vi "Main.vi"(11 "Module Admin":refnum<class "Delacor_lib_QMH_Module Admin.lvclass">) -> ()   [LabVIEW 2020, in "Rename As Application UI.lvlib"]
doc: "This template is based off of the Queued Message Handler design pattern and the Queued Message Handler project template that ships with LabVIEW.\n\nThe main difference is that the queue is private to this module and communication between modules is performed via Broadcast and Request events.\n\nRequest events are wrapped in public API methods and are handled in the Event Handling Loop (EHL) of this VI. Any module can register for Broadcast events sent by this module. The EHL generates messages based on user interface actions.\n\nThe Message Handling Loop (MHL) processes messages generated by the EHL, or by other messages. The messages are string values, so new messages can be added easily to the Message Cases case structure in the MHL. Each message cluster can also provide an optional value for Message Data, which is a variant that can be converted to whatever message-specific data is required.\n_____\nBased on DQMH Project Template 6.1.0.94."
uses:
  Rename As Application UI.lvlib
  <vilib>/Delacor/Delacor QMH/Libraries/Module Admin_class/Delacor_lib_QMH_Module Admin.lvclass
  Module Data--cluster.ctl
  Configuration/Configuration--cluster.ctl
  <vilib>/Delacor/Delacor QMH/Libraries/Message Queue_class/Delacor_lib_QMH_Message Queue.lvclass/Delacor_lib_QMH_Message Queue.ctl
  Stop Argument--cluster.ctl
  <vilib>/Utility/miscctls.llb/LVPointTypeDef.ctl
  <vilib>/Delacor/Delacor QMH/Libraries/Module Admin_class/Delacor_lib_QMH_Module Admin.lvclass/Delacor_lib_QMH_Module Admin.ctl
  <vilib>/Delacor/Delacor QMH/Libraries/Message Queue_class/Delacor_lib_QMH_Enqueue Message (Single).vi
  <vilib>/Delacor/Delacor QMH/Libraries/Module Admin_class/Delacor_lib_QMH_Get External Launch.vi
  <vilib>/Utility/error.llb/Error Cluster From Error Code.vi
  <vilib>/ErrorRing/Error Ring.xnode
  <vilib>/Delacor/Delacor QMH/Libraries/Message Queue_class/Delacor_lib_QMH_Message Queue.lvclass
  <vilib>/Peloton/Pelobuttons/Pelobuttons_lib_Pelobuttons.lvlib
  Configuration/Configuration.lvlib
  <vilib>/Peloton/Peloton Config/Libraries/DCFG Framework/Peloton_DCFG Framework.lvlib
  Rename As Application Shared/Rename as Application Shared.lvlib
  Motherboard loading/Motherboard loading.lvlib
panel:
  in  "STOP":bool
  in  "Detecting speed":dbl caption="Detecting spedd" format="%#_6pms"
  in  "Start Acquisition":bool
  out "Waveform Chart":i32(graph)
  out "version":string
  in  "About":bool
  in  "Configuration":bool
  in  "Random Path":path
  out "error out":errorcluster
  in  "Simulate MHL Error":bool
  in  "Simulate EHL Error":bool
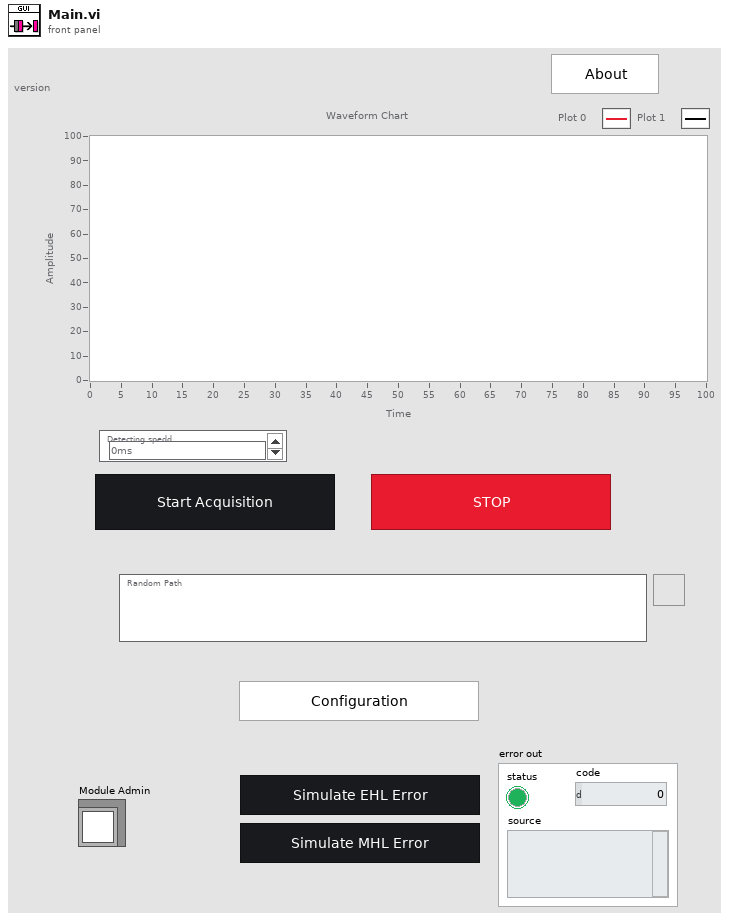
[diagram p1: front panel]
types:
  T1 = typedef "Rename As Application UI.lvlib/Request Events--cluster.ctl" = cluster{"Stop Module":refnum<user-event>, "Show Panel":refnum<user-event>, "Hide Panel":refnum<user-event>, "Get Module Execution Status":refnum<user-event>, "Show Diagram":refnum<user-event>}
  T2 = typedef "Peloton_DCFG Framework.lvlib/Broadcast Events--cluster.ctl" = cluster{"Module Did Init":refnum<user-event>, "Status Updated":refnum<user-event>, "Error Reported":refnum<user-event>, "Module Did Stop":refnum<user-event>, "Update Module Execution Status":refnum<user-event>, "View Changed":refnum<user-event>, "Configuration Updated":refnum<user-event>, "Page Error Received":refnum<user-event>, "Page List Updated":refnum<user-event>, "Defaults Applied":refnum<user-event>, "Main Window Closed":refnum<user-event>}
  T3 = typedef "Motherboard loading.lvlib/Broadcast Events--cluster.ctl" = cluster{"Module Did Init":refnum<user-event>, "Status Updated":refnum<user-event>, "Error Reported":refnum<user-event>, "Module Did Stop":refnum<user-event>, "Update Module Execution Status":refnum<user-event>, "CPU Loading updated":refnum<user-event>}
  T4 = typedef "Rename As Application UI.lvlib/Module Data--cluster.ctl" = cluster{"UI Configuration":T5}
  T5 = typedef "Rename As Application UI.lvlib/Configuration.lvlib/Configuration--cluster.ctl" = cluster{"Random Path":path}
  T6 = enum32{"invalid lock state", "Not Locked", "Locked (No Password)", "Password-protected"}
  T7 = typedef "Rename As Application UI.lvlib/Stop Argument--cluster.ctl" = cluster{"Origin":string, "Exit via Stop Module Req?":bool, "Wait for Module to stop?":bool}
  T8 = typedef "LVPointTypeDef.ctl" = cluster{"Horizontal":i16, "Vertical":i16}
  T9 = enum32{"Invalid", "Standard", "Closed", "Hidden", "Minimized", "Maximized"}
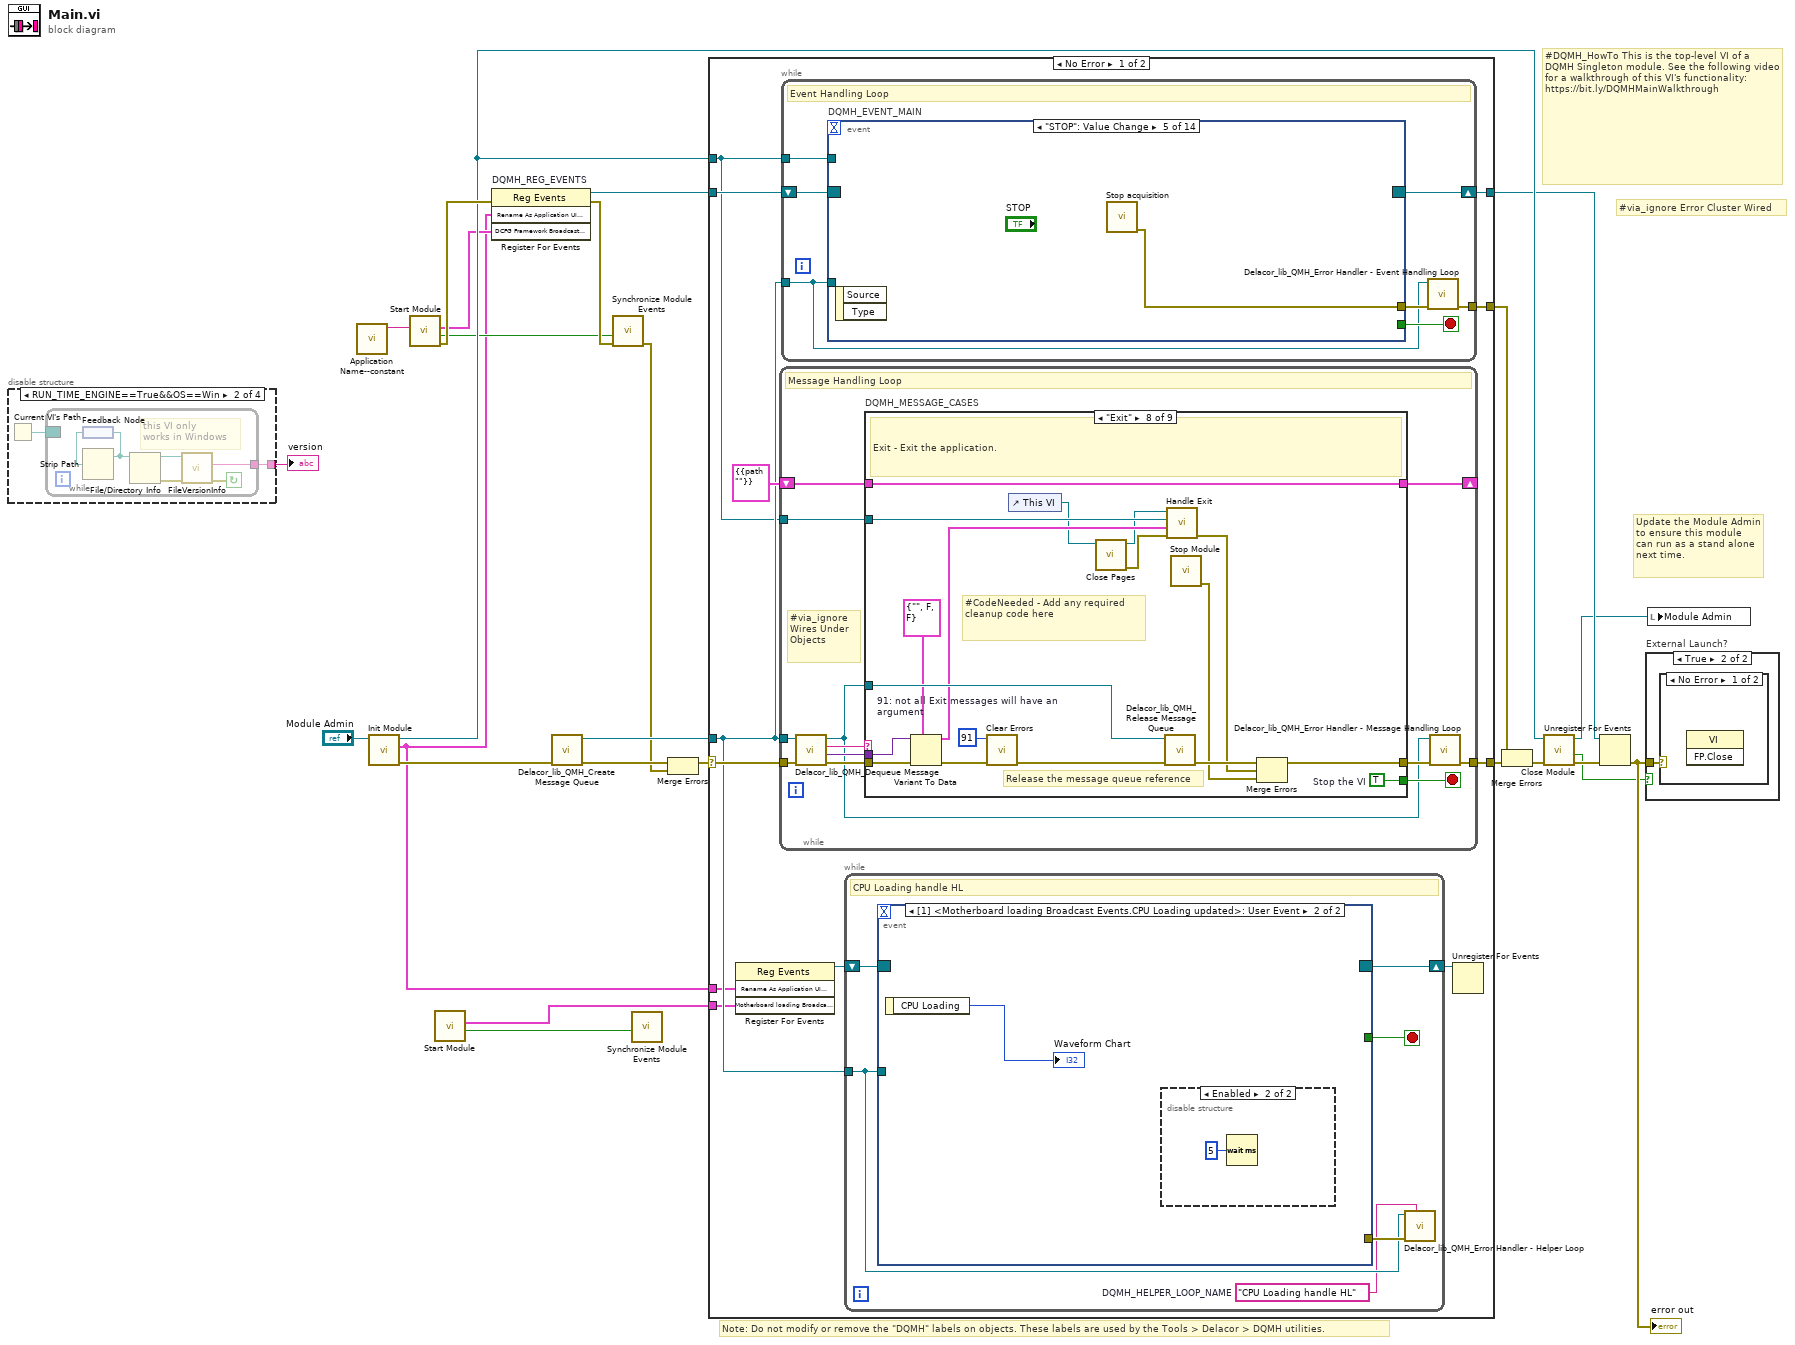
[diagram p0: block diagram]
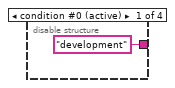
[diagram p2: hidden frame]
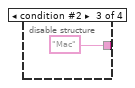
[diagram p3: hidden frame]
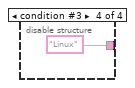
[diagram p4: hidden frame]
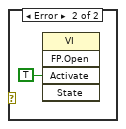
[diagram p6: hidden frame]
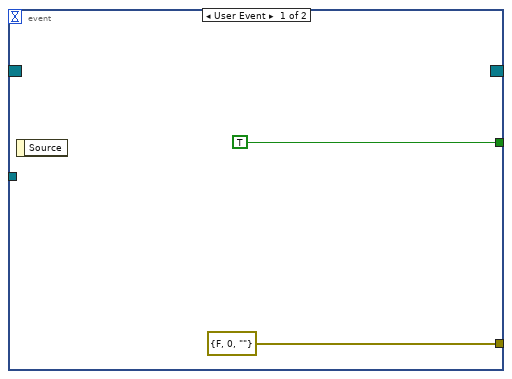
[diagram p7: hidden frame]
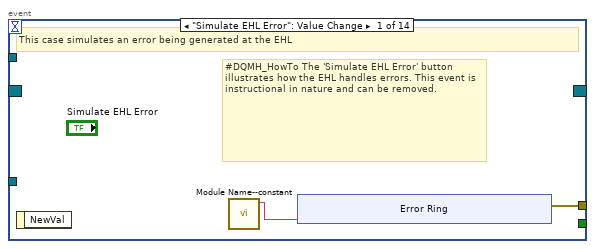
[diagram p9: hidden frame]
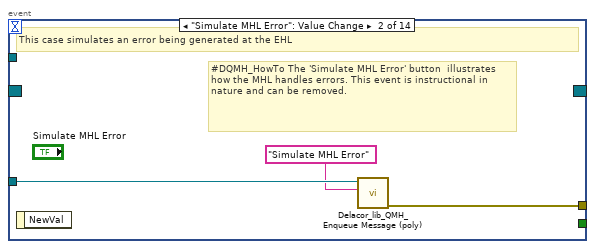
[diagram p10: hidden frame]
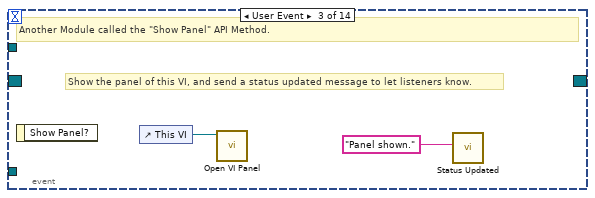
[diagram p11: hidden frame]
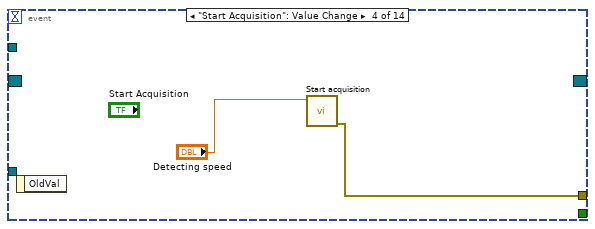
[diagram p12: hidden frame]
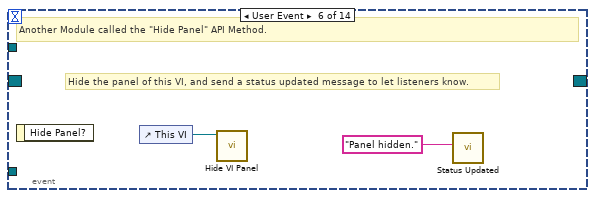
[diagram p13: hidden frame]
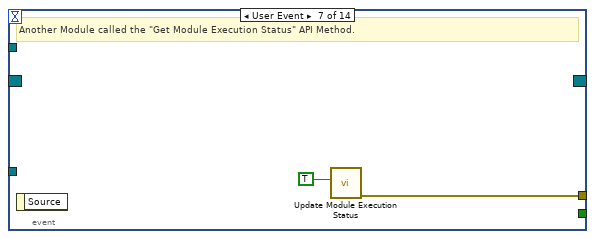
[diagram p14: hidden frame]
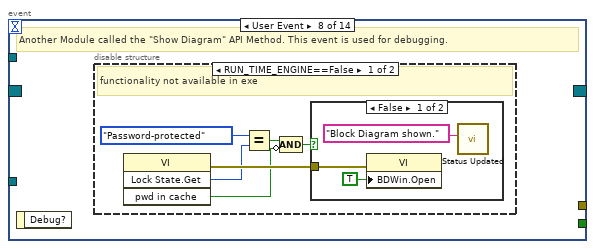
[diagram p15: hidden frame]
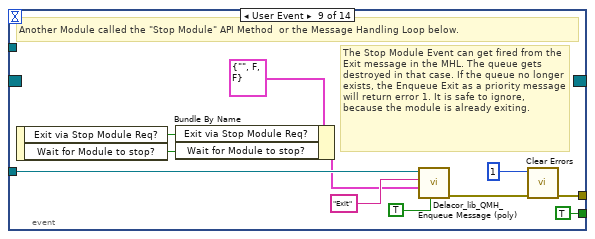
[diagram p18: hidden frame]
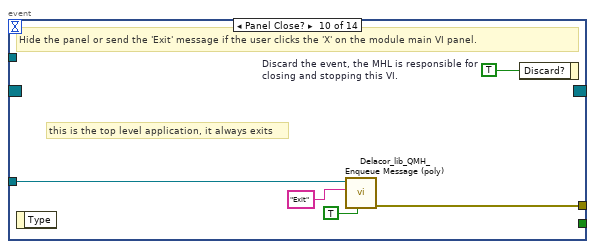
[diagram p19: hidden frame]
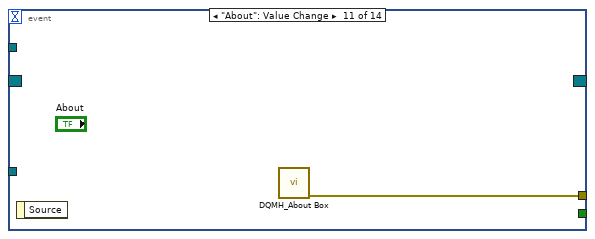
[diagram p20: hidden frame]
diagram:
  # "#via_ignore Error Cluster Wired"
  # "#DQMH_HowTo This is the top-level VI of a DQMH Singleton module. See the following video for a walkthrough of this VI's functionality: https://bit.ly/DQMHMainWalkthrough"
  # "Note: Do not modify or remove the \"DQMH\" labels on objects. These labels are used by the Tools > Delacor > DQMH utilities."
  # "Update the Module Admin to ensure this module can run as a stand alone next time."
  n1 = disable-structure "Conditional Disable Structure" shown="RUN_TIME_ENGINE==True&&OS==Win" {
    disable-tunnel: ["development" w27 "Mac" "Linux"] -> w4
    frame condition #0 (active) {
    }
    frame condition #1 {
      n2 = Current VI's Path() -> (path=w28:path)
      n3 = while {
        border: w28 -> [_]
        tunnel: [w29] -> w27
        stop <- w33 continue-if-true
        # "this VI only \nworks in Windows"
        n4 = feedback #1() -> (w32:path)
        n5 = Strip Path(path=w32) -> (stripped path=w31:path)  [unwired: 1 out]
        n6 = feedback-in #1(w31) -> ()
        n7 = File/Directory Info(path=w31) -> (path out=w30:path, error out=w34:errorcluster)  [unwired: 1 in, 5 out]
        n8 = call <vilib>:"FileVersionInfo.vi"("error in (no error)"=w34, "Application Path in"=w30) -> ("error out"=w33:errorcluster, "File Version Info"=w29:string)  [unwired: 6 in, 2 out]
      }
    }
    frame condition #2 {
    }
    frame condition #3 {
    }
  }
  "version" <- w4
  n9 = call "Application Name--constant.vi"() -> ("Application Name"=w9:string)  [unwired: 11 in]
  n10 = call "Init Module.vi"("Singleton Module Admin in"="Module Admin") -> ("error out"=w23:errorcluster, "Rename As Application UI Request Events"=w2:T1, "Singleton Module Admin out"=w16:refnum<class "Delacor_lib_QMH_Module Admin.lvclass">)  [unwired: 8 in]
  n11 = call <vilib>:"Start Module.vi"("Application Name"=w9) -> ("error out"=w25:errorcluster, "Wait for Event Sync?"=w6:bool, "DCFG Framework Broadcast Events"=w5:T2)  [unwired: 7 in, 1 out]
  n12 = call <vilib>:"Start Module.vi"() -> ("Wait for Event Sync?"=w3:bool, "Motherboard loading Broadcast Events"=w1:T3)  [unwired: 8 in, 2 out]
  n13 = register-events "DQMH_REG_EVENTS"(error in=w25, w2, w5) -> (reference out=w14:refnum<event-registration>, error out=w8:errorcluster)  [unwired: 1 in]
  n14 = call <vilib>:"Delacor_lib_QMH_Create Message Queue.vi"("error in"=w23) -> ("error out"=w18:errorcluster, "Message Queue"=w13:refnum<class "Delacor_lib_QMH_Message Queue.lvclass">)  [unwired: 9 in]
  n15 = call <vilib>:"Synchronize Module Events.vi"("error in (no error)"=w8, "Wait for Event Sync?"=w6) -> ("error out"=w7:errorcluster)  [unwired: 9 in]
  n16 = call <vilib>:"Synchronize Module Events.vi"("Wait for Event Sync?"=w3) -> ()  [unwired: 10 in, 1 out]
  n17 = Merge Errors(w18, w7) -> (w17:errorcluster)
  n18 = case shown="No Error" w17 {
    selector: w17 -> [w46 w235]
    tunnel: [w48 w234] -> w24
    tunnel: [w45 w240] -> w15
    tunnel: w14 -> [w43 w240]
    tunnel: w13 -> [w42 w233]
    tunnel: [w47 _] -> w21
    tunnel: w16 -> [w41 w236]
    tunnel: w2 -> [w40 _]
    tunnel: w1 -> [w37 _]
    frame No Error {
      n19 = register-events ("DQMH_HELPER_REGFOREVENTS")(w40, w37) -> (reference out=w38:refnum<event-registration>)  [unwired: 2 in, 1 out]
      n20 = while {
        tunnel: w42 -> [w127]
        shift-right: [w131] -> _
        shift-left: T4 {"UI Configuration"={"Random Path"=path ""}} ("Data Cluster") -> [w132]
        tunnel: w46 -> [w135]
        tunnel: [w133] -> w48
        tunnel: w41 -> [w125]
        stop <- w130 stop-if-true
        # "#via_ignore Wires Under Objects"
        # "Message Handling Loop"
        n21 = call-dynamic "Delacor_lib_QMH_Dequeue Message.vi"("error in"=w135, "Message Queue in"=w127) -> ("error out"=w134:errorcluster, "Message Data"=w128:variant, "Message"=w129:string, "Message Queue out"=w126:refnum<class "Delacor_lib_QMH_Message Queue.lvclass">)  [unwired: 6 in]
        n22 = case "DQMH_MESSAGE_CASES" shown="\"Exit\"" w129 {
          selector: w129 -> [_ _ _ _ _ _ _ _ w220]
          tunnel: w126 -> [_ _ _ _ _ _ w187 w211 _]
          tunnel: w134 -> [w155 w159 w167 w170 w172 w177 w194 w217 w222]
          tunnel: [w154 w159 w164 w169 w172 w176 w190 w214 w223] -> w136
          tunnel: w132 -> [w145 w158 w166 w168 w171 w174 w189 w210 w221]
          tunnel: [w144 w158 w165 w168 w171 w174 w189 w210 w221] -> w131
          tunnel: [_ _ _ _ _ _ _ w209 _] -> w130
          tunnel: w128 -> [_ _ w163 _ _ _ w188 w218 _]
          tunnel: w125 -> [w146 _ _ _ _ _ w186 w205 _]
          frame "Initialize" {
            # "#CodeNeeded - Initialize the appearance of the front panel."
            # "Initialize - Any operation that needs to be done before the module can receive messages. Synchronize Caller Events.vi will inform Start Module.vi that the module has launched and is ready to receive messages. Module Did Init.vi will broadcast that the module initialized."
            n23 = call "Synchronize Caller Events.vi"("error in (no error)"=w155, "Singleton Module Admin in"=w146) -> ("error out"=w139:errorcluster, "Singleton Module Admin out"=w141:refnum<class "Delacor_lib_QMH_Module Admin.lvclass">)  [unwired: 8 in]
            n24 = property on="Property Node" class="Module Admin"(reference=w141) -> ("Accessors:External Launch"=w150:bool)  [unwired: 1 in, 2 out]
            n25 = flat-sequence {
              tunnel: w139 -> [_]
              frame #0 {
                n26 = call <vilib>:"Brand UI - FP.vi"() -> ()  [unwired: 12 in]
              }
            }
            n27 = call "Add Pages.vi"("error in (no error)"=w139) -> ("latest data"=w138:T5)  [unwired: 9 in, 1 out]
            n28 = Select(t=T9."Hidden" ("State"), s=w150, f=T9."Standard" ("State")) -> (s? t:f=w147:T9)
            n29 = Unbundle By Name(w138) -> ("Random Path"=w137:path)
            n30 = call "Module Name--constant.vi"() -> ("Module Name"=w153:string)  [unwired: 11 in]
            n31 = property on="Property Node" class="VI"("Front Panel.Title"=w153) -> (reference out=w152:refnum<vi>, error out=w157:errorcluster)  [unwired: 2 in]
            n32 = call "Module Name--constant.vi"() -> ("Module Name"=w142:string)  [unwired: 11 in]
            n33 = local write "Random Path"(w137) -> ()
            n34 = Bundle By Name(cluster=w145, "UI Configuration"=w138) -> (w144:T4)
            n35 = invoke on="Invoke Node" class="VI" method="FP.Open"(reference=w152, error in=w157, "State"=w147) -> (reference out=w151:refnum<vi>, error out=w156:errorcluster)  [unwired: 2 in, 3 out]
            n36 = call "Module Did Init.vi"("error in (no error)"=w139, "Initialized?"=TRUE, "Origin"=w142) -> ("error out"=w154:errorcluster)  [unwired: 8 in]
            n37 = invoke on="Invoke Node" class="VI" method="FP.Center"(reference=w151, error in=w156) -> ()  [unwired: 1 in, 3 out]
            n38 = property on="Pane" class="Pane"("Origin"=T8 {"Horizontal"=0, "Vertical"=0}) -> ()  [unwired: 2 in, 2 out]
          }
          frame "---Module Specific---" {
            # "Separator -- The following cases handle messages specific to this Module."
          }
          frame "Configuration Updated" {
            # "The Configuration Editor has broadcasted that the Configuration has been updated"
            n39 = Variant To Data(error in=w167, type=T5 {"Random Path"=path ""} ("UI Configuration"), Variant=w163) -> (data=w161:T5, error out=w164:errorcluster)
            n40 = Unbundle By Name(w161) -> ("Random Path"=w160:path)
            n41 = Bundle By Name(cluster=w166, "UI Configuration"=w161) -> (w165:T4)
            n42 = local write "Random Path"(w160) -> ()
          }
          frame "---Copy This Frame---" {
            # "Duplicate this frame when creating new messages.  Change this comment in the duplicated frame to describe this message."
            n43 = Merge Errors(w170) -> (w169:errorcluster)
          }
          frame "---Exit and Error Handling---" {
            # "Separator - The following cases handle errors and exit messages."
          }
          frame "Simulate MHL Error" {
            # "#DQMH_HowTo The 'Simulate MHL Error' button  illustrates how the MHL handles errors. This event is instructional in nature and can be removed."
            # "Simulate an error occurring at the MHL"
            n44 = call "Module Name--constant.vi"() -> ("Module Name"=w173:string)  [unwired: 11 in]
            n45 = xnode ("Error Ring")("parameter 0"=w173) -> ("error out"=w175:errorcluster)
            n46 = Merge Errors(w177, w175) -> (w176:errorcluster)
          }
          frame "Error" {
            # "#CodeRecommended - If you ever change the name of this \"Error\" message, you'll need to update the name in the Check Loop Error.vi as well."
            # "#CodeRecommended - If the module is running in standalone mode (External Launch = FALSE), this code will pop up an error dialog and call the 'Exit' message if an error occurs. Add more fine-grained error handling here."
            # "Error - Check the error message data and respond accordingly. This message is sent by the \"Error Handler\" VIs at the end of each loop in this application."
            n47 = property on="Property Node" class="Module Admin"(reference=w186) -> ("Accessors:External Launch"=w185:bool)  [unwired: 1 in, 2 out]
            n48 = Variant To Data(error in=w194, type=errorcluster {"status"=FALSE, "code"=0, "source"=""} ("error constant"), Variant=w188) -> (data=w195:errorcluster, error out=w192:errorcluster)
            n49 = call "Error Reported.vi"("Error"=w195) -> ()  [unwired: 10 in, 1 out]
            n50 = case shown="False" w185 {
              tunnel: [w200 _] -> w191
              tunnel: w187 -> [w198 _]
              tunnel: w195 -> [w199 _]
              frame False {
                # "If the module is running standalone, then pop up an error dialog and call the \"Exit\" message."
                n51 = call <vilib>:"Simple Error Handler.vi"("error in (no error)"=w199) -> ()  [unwired: 4 in, 5 out]
                n52 = call-poly <vilib>:"Delacor_lib_QMH_Enqueue Message (poly).vi"("Priority Message? (F)"=TRUE, "Message"="Exit", "Message Queue in"=w198) -> ("error out"=w200:errorcluster)  [unwired: 7 in, 1 out]
              }
              frame True {
                # "If the module was launched externally, calling the Error Reported broadcast VI is the only action performed by the \"Error\" message. The module's caller can then process the error appropriately."
              }
            }
            n53 = Merge Errors(w192, w191) -> (w190:errorcluster)
            n54 = local write "error out"(w190) -> ()
          }
          frame "Exit" {
            w208 = 91  # 91: not all Exit messages will have an argument
            w209 = TRUE  # Stop the VI
            # "Release the message queue reference"
            # "#CodeNeeded - Add any required cleanup code here"
            # "Exit - Exit the application."
            n55 = Variant To Data(error in=w217, type=T7 {"Origin"="", "Exit via Stop Module Req?"=FALSE, "Wait for Module to stop?"=FALSE} ("Stop Argument"), Variant=w218) -> (data=w206:T7, error out=w213:errorcluster)
            n56 = call <vilib>:"Clear Errors.vi"("error in (no error)"=w213, "specific error code to clear (0: all)"=w208) -> ("error out"=w216:errorcluster)  [unwired: 4 in, 1 out]
            n57 = control-ref of="This VI"() -> (w203:refnum<vi>)
            n58 = call "Close Pages.vi"("Calling VI in"=w203) -> ("error out"=w204:errorcluster, "Calling VI out"=w202:refnum<vi>)  [unwired: 9 in]
            n59 = call-dynamic "Delacor_lib_QMH_Release Message Queue.vi"("error in"=w216, "Message Queue"=w211) -> ("error out"=w215:errorcluster)  [unwired: 9 in]
            n60 = call "Handle Exit.vi"("error in (no error)"=w204, "Stop Argument"=w206, "Admin in"=w205, "VI reference"=w202) -> ("error out"=w212:errorcluster)  [unwired: 6 in, 1 out]
            n61 = call "Stop Module.vi"() -> ("error out"=w201:errorcluster)  [unwired: 11 in]
            n62 = Merge Errors(w215, w212, w201) -> (w214:errorcluster)
          }
          frame Default {
            # "'Default' case only runs if there is a message that isn't defined in any of the other cases.  Output a programming error."
            n63 = call "Module Name--constant.vi"() -> ("Module Name"=w219:string)  [unwired: 11 in]
            n64 = xnode ("Error Ring")("parameter 0"=w220, "parameter 1"=w219) -> ("error out"=w224:errorcluster)
            n65 = Merge Errors(w222, w224) -> (w223:errorcluster)
          }
        }
        n66 = call-dynamic "Delacor_lib_QMH_Error Handler - Message Handling Loop.vi"("error in"=w136, "Message Queue in"=w126) -> ("dup error in"=w133:errorcluster)  [unwired: 8 in, 1 out]
      }
      n67 = while {
        tunnel: w42 -> [w59]
        shift-right: [w62] -> w45
        shift-left: w43 -> [w63]
        tunnel: [w64] -> w47
        tunnel: w41 -> [w60]
        stop <- w61 stop-if-true
        # "Event Handling Loop"
        n68 = event "DQMH_EVENT_MAIN" shown="[4] \"STOP\": Value Change" {
          selector: w63 -> [_ _ _ _ _ _ _ _ _ _ _ _ _ _]
          dyn-events: [_ _ _ _ _ _ _ _ _ _ _ _ _ _] -> w62
          timeout: _ -> [_ _ _ _ _ _ _ _ _ _ _ _ _ _]
          tunnel: [_ _ _ _ _ _ _ _ TRUE ("Discard?") _ _ _ _ _] -> w61
          tunnel: w59 -> [_ w76 _ _ _ _ _ _ w102 w109 _ _ w115 _]
          tunnel: [w67 w77 _ w81 w82 _ w86 _ w105 w111 w112 _ w114 w123] -> w65
          tunnel: w60 -> [_ _ _ _ _ _ _ _ _ _ _ _ _ _]
          event "Simulate EHL Error": Value Change {
            # "#DQMH_HowTo The 'Simulate EHL Error' button  illustrates how the EHL handles errors. This event is instructional in nature and can be removed."
            # "This case simulates an error being generated at the EHL"
            n69 = event-data() -> ()  [unwired: 1 in, 1 out]
            n70 = call "Module Name--constant.vi"() -> ("Module Name"=w66:string)  [unwired: 11 in]
            n71 = xnode ("Error Ring")("parameter 0"=w66) -> ("error out"=w67:errorcluster)
          }
          event "Simulate MHL Error": Value Change {
            # "#DQMH_HowTo The 'Simulate MHL Error' button  illustrates how the MHL handles errors. This event is instructional in nature and can be removed."
            # "This case simulates an error being generated at the EHL"
            n72 = event-data() -> ()  [unwired: 1 in, 1 out]
            n73 = call-poly <vilib>:"Delacor_lib_QMH_Enqueue Message (poly).vi"("Message"="Simulate MHL Error", "Message Queue in"=w76) -> ("error out"=w77:errorcluster)  [unwired: 8 in, 1 out]
          }
          event User Event {
            # "Show the panel of this VI, and send a status updated message to let listeners know."
            # "Another Module called the \"Show Panel\" API Method."
            n74 = event-data() -> ()  [unwired: 1 in, 1 out]
            n75 = control-ref of="This VI"() -> (w79:refnum<vi>)
            n76 = call "Open VI Panel.vi"("VI"=w79) -> ()  [unwired: 10 in, 1 out]
            n77 = call "Status Updated.vi"("Status"="Panel shown." ("format string")) -> ()  [unwired: 10 in, 1 out]
          }
          event "Start Acquisition": Value Change {
            n78 = event-data() -> ()  [unwired: 1 in, 1 out]
            n79 = call "Start acquisition.vi"("Detecting speed"="Detecting speed") -> ("error out"=w81:errorcluster)  [unwired: 9 in, 1 out]
          }
          event "STOP": Value Change {
            n80 = event-data() -> ()  [unwired: 1 in, 2 out]
            n81 = call "Stop acquisition.vi"() -> ("error out"=w82:errorcluster)  [unwired: 11 in]
          }
          event User Event {
            # "Hide the panel of this VI, and send a status updated message to let listeners know."
            # "Another Module called the \"Hide Panel\" API Method."
            n82 = event-data() -> ()  [unwired: 1 in, 1 out]
            n83 = control-ref of="This VI"() -> (w84:refnum<vi>)
            n84 = call "Hide VI Panel.vi"("VI"=w84) -> ()  [unwired: 10 in, 1 out]
            n85 = call "Status Updated.vi"("Status"="Panel hidden." ("format string")) -> ()  [unwired: 10 in, 1 out]
          }
          event User Event {
            # "Another Module called the \"Get Module Execution Status\" API Method."
            n86 = event-data() -> ()  [unwired: 1 in, 1 out]
            n87 = call "Update Module Execution Status.vi"("Running?"=TRUE) -> ("error out"=w86:errorcluster)  [unwired: 10 in]
          }
          event User Event {
            # "Another Module called the \"Show Diagram\" API Method. This event is used for debugging."
            n88 = event-data() -> ()  [unwired: 1 in, 1 out]
            n89 = disable-structure shown="RUN_TIME_ENGINE==False" {
              frame condition #0 (active) {
                # "functionality not available in exe"
                n90 = invoke on="Invoke Node" class="VI" method="Lock State.Get"() -> (error out=w92:errorcluster, "Get Lock State"=w91:T6, "pwd in cache"=w88:bool)  [unwired: 4 in, 1 out]
                n91 = Equal?(x=T6."Password-protected", y=w91) -> (x = y?=w89:bool)
                n92 = Compound Arithmetic op=AND(w89, invert w88) -> (w87:bool)
                n93 = case shown="False" w87 {
                  tunnel: w92 -> [w95 _]
                  frame False {
                    n94 = property on="Property Node" class="VI"(error in=w95, "BDWin.Open"=TRUE ("Block Diagram Window:Open")) -> ()  [unwired: 1 in, 2 out]
                    n95 = call "Status Updated.vi"("Status"="Block Diagram shown." ("format string")) -> ()  [unwired: 10 in, 1 out]
                  }
                  frame True {
                    # "Password-protected VI, and the password is not in the cache. Do not show the diagram."
                  }
                }
              }
              frame condition #1 {
              }
            }
          }
          event User Event {
            # "The Stop Module Event can get fired from the Exit message in the MHL. The queue gets destroyed in that case. If the queue no longer exists, the Enqueue Exit as a priority message will return error 1. It is safe to ignore, because the module is already exiting."
            # "Another Module called the \"Stop Module\" API Method  or the Message Handling Loop below."
            n96 = event-data() -> ("Exit via Stop Module Req?"=w98:bool, "Wait for Module to stop?"=w97:bool)  [unwired: 1 in]
            n97 = Bundle By Name(cluster=T7 {"Origin"="", "Exit via Stop Module Req?"=FALSE, "Wait for Module to stop?"=FALSE} ("Stop Argument"), "Exit via Stop Module Req?"=w98, "Wait for Module to stop?"=w97) -> (w96:T7)
            n98 = call-poly <vilib>:"Delacor_lib_QMH_Enqueue Message (poly).vi"("Priority Message? (F)"=TRUE, "Message Data"=w96, "Message"="Exit", "Message Queue in"=w102) -> ("error out"=w106:errorcluster)  [unwired: 6 in, 1 out]
            n99 = call <vilib>:"Clear Errors.vi"("error in (no error)"=w106, "specific error code to clear (0: all)"=1) -> ("error out"=w105:errorcluster)  [unwired: 4 in, 1 out]
          }
          event Panel Close? {
            w110 = TRUE  # Discard the event, the MHL is responsible for closing and stopping this VI.
            # "this is the top level application, it always exits"
            # "Hide the panel or send the 'Exit' message if the user clicks the 'X' on the module main VI panel."
            n100 = event-data() -> ()  [unwired: 1 in, 1 out]
            n101 = call-poly <vilib>:"Delacor_lib_QMH_Enqueue Message (poly).vi"("Priority Message? (F)"=TRUE, "Message"="Exit", "Message Queue in"=w109) -> ("error out"=w111:errorcluster)  [unwired: 7 in, 1 out]
            n102 = event-data ("Event Filter Node")("Discard?"=w110) -> ()  [unwired: 1 in, 1 out]
          }
          event "About": Value Change {
            n103 = event-data() -> ()  [unwired: 1 in, 1 out]
            n104 = call <vilib>:"DQMH_About Box.vi"() -> ("error out"=w112:errorcluster)  [unwired: 11 in]
          }
          event "Configuration": Value Change {
            n105 = event-data() -> ()  [unwired: 1 in, 1 out]
            n106 = call <vilib>:"Show Panel.vi"() -> ()  [unwired: 11 in, 1 out]
          }
          event User Event {
            # "The Configuration Editor has broadcasted that the Configuration has been updated"
            n107 = event-data() -> ("New Data"=w118:variant, "Name"=w117:string)  [unwired: 1 in]
            n108 = call "Handle Configuration Updated.vi"("Name"=w117, "New Data"=w118) -> ("Addressed to this Module"=w116:bool, "Latest Data"=w113:T5)  [unwired: 7 in, 1 out]
            n109 = case shown="True" w116 {
              tunnel: w115 -> [_ w122]
              tunnel: [_ w121] -> w114
              tunnel: w113 -> [_ w120]
              frame False {
              }
              frame True {
                n110 = call-poly <vilib>:"Delacor_lib_QMH_Enqueue Message (poly).vi"("Message Data"=w120, "Message"="Configuration Updated", "Message Queue in"=w122) -> ("error out"=w121:errorcluster)  [unwired: 7 in, 1 out]
              }
            }
          }
          event "Random Path": Value Change {
            n111 = event-data() -> ("NewVal"=w124:path)  [unwired: 1 in]
            n112 = call "Update Configuration.vi"("Random Path"=w124) -> ("error out"=w123:errorcluster)  [unwired: 10 in]
          }
        }
        n113 = call-dynamic "Delacor_lib_QMH_Error Handler - Event Handling Loop.vi"("error in"=w65, "Message Queue in"=w59) -> ("dup error in"=w64:errorcluster)  [unwired: 8 in, 1 out]
      }
      n114 = while "DQMH_HELPER_LOOP" {
        shift-right: [w53] -> w39
        shift-left: w38 -> [w54]
        tunnel: w42 -> [w50]
        stop <- w52 stop-if-true
        w49 = "CPU Loading handle HL"  # DQMH_HELPER_LOOP_NAME
        # "CPU Loading handle HL"
        n115 = event "DQMH_HELPER_EVENT_STRUCTURE" shown="[1] <Motherboard loading Broadcast Events.CPU Loading updated>: User Event" {
          selector: w54 -> [_ _]
          dyn-events: [_ _] -> w53
          timeout: _ -> [_ _]
          tunnel: [TRUE _] -> w52
          tunnel: [errorcluster {"status"=FALSE, "code"=0, "source"=""} ("error constant") _] -> w51
          tunnel: w50 -> [_ _]
          event User Event {
            n116 = event-data() -> ()  [unwired: 1 in, 1 out]
          }
          event User Event {
            n117 = event-data() -> ("CPU Loading"=→"Waveform Chart":i32)  [unwired: 1 in]
            n118 = disable-structure shown="Enabled" {
              frame Disabled {
              }
              frame Enabled {
                n119 = Wait (ms)(milliseconds to wait=u32 5) -> ()  [unwired: 1 out]
              }
            }
          }
        }
        n120 = call-dynamic "Delacor_lib_QMH_Error Handler - Helper Loop.vi"("Error Debug"=w49, "error in"=w51, "Message Queue in"=w50) -> ()  [unwired: 7 in, 2 out]
      }
      n121 = Unregister For Events(event registration refnum=w39) -> ()  [unwired: 1 in, 1 out]
    }
    frame Error {
      # "Synchronize Caller Events.vi will inform Start Module.vi that the module has launched and will let the code calling Start Module.vi register for broadcasts and would permit the caller receive the broadcast that an error occurred at launch time."
      n122 = call-dynamic "Delacor_lib_QMH_Release Message Queue.vi"("error in"=w235, "Message Queue"=w233) -> ("error out"=w234:errorcluster)  [unwired: 9 in]
      n123 = call "Synchronize Caller Events.vi"("Singleton Module Admin in"=w236) -> ("error out"=w241:errorcluster)  [unwired: 9 in, 1 out]
      n124 = call "Module Name--constant.vi"() -> ("Module Name"=w239:string)  [unwired: 11 in]
      n125 = Format Into String(format string="An error occurred during initialization. %s is no longer running.", w239) -> (resulting string=w237:string)  [unwired: 2 in, 1 out]
      n126 = Merge Errors(w234, w241) -> (w242:errorcluster)
      n127 = call <vilib>:"Calling Module Error on Init.vi"() -> ()  [unwired: 11 in, 1 out]
      n128 = call "Error Reported.vi"("Additional Information"=w237, "Error"=w242) -> ()  [unwired: 9 in, 1 out]
    }
  }
  n129 = Merge Errors(w21, w24) -> (w20:errorcluster)
  n130 = call "Close Module.vi"("error in (no error)"=w20, "Module Admin in"=w16) -> ("error out"=w22:errorcluster, "External Launch"=w10:bool, "Module Admin out"=w11:refnum<class "Delacor_lib_QMH_Module Admin.lvclass">)  [unwired: 7 in]
  n131 = Unregister For Events(event registration refnum=w15, error in=w22) -> (error out=w19:errorcluster)
  "error out" <- w19
  n132 = case "External Launch?" shown="True" w10 {
    tunnel: w19 -> [_ w243]
    frame False {
    }
    frame True {
      n133 = case shown="No Error" w243 {
        frame No Error {
          n134 = invoke class="VI" method="FP.Close"() -> ()  [unwired: 3 in, 3 out]
        }
        frame Error {
          n135 = invoke on="Invoke Node" class="VI" method="FP.Open"("Activate"=TRUE ("Activate?")) -> ()  [unwired: 4 in, 5 out]
        }
      }
    }
  }
  n136 = local write "Module Admin"(w11) -> ()
